vi "Read Selected Channel.vi"(10 "Channel Name":string, 11 "Waveform In":waveform(dbl)[](array[waveform])) -> (3 "Selected Channel":waveform(dbl))   [LabVIEW 2019, in "Variant Parser.lvlib" / "Variant Parser.lvclass"]
uses:
  Library/Variant Parser.lvclass
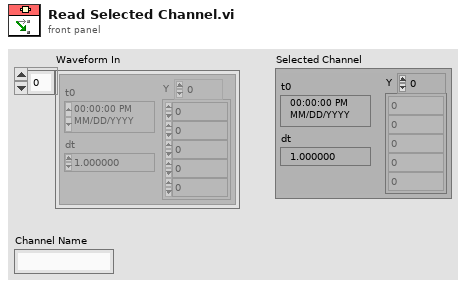
[diagram p1: front panel]
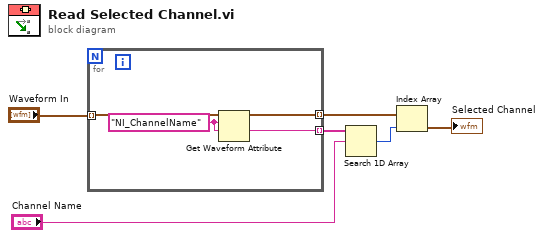
[diagram p0: block diagram]
diagram:
  n1 = for {
    tunnel: "Waveform In" -> [w10] mode=indexing
    tunnel: [w8] -> w4 mode=indexing
    tunnel: [w7] -> w3 mode=indexing
    w9 = "NI_ChannelName" ("name")
    n2 = Get Waveform Attribute(5:w9, 6:w9, 7:w10) -> (1:w7:string, 3:w8:waveform(dbl))  [unwired: 1 in, 2 out]
  }
  n3 = Search 1D Array(1D array=w3, element="Channel Name") -> (index of element=w5:i32)  [unwired: 1 in]
  n4 = Index Array(array=w4, index=w5) -> (element=→"Selected Channel":waveform(dbl))
